vi "compressor_getenablstate.vi"(0 "CompressorDevRef":T1={"DevStatus"={"status"=FALSE, "code"=0, "source"=""}, "DigitalInputDevRef"={"DevStatus"={"status"=FALSE, "code"=0, "source"=""}, "DIO Channel"=enum."DIO 1", "Digital Module"=enum."Digital Module 1"}, "RelayDevRef"={"DevStatus"={"status"=FALSE, "code"=0, "source"=""}, "Relay Channel"=enum."Invalid", "Digital Module"=enum."Digital Module 1", "Relay Direction"=enum."Both directions"}}, 11 "error in (no error)":errorcluster) -> (4 "CompressorDevRef":T1={"DevStatus"={"status"=FALSE, "code"=0, "source"=""}, "DigitalInputDevRef"={"DevStatus"={"status"=FALSE, "code"=0, "source"=""}, "DIO Channel"=enum."DIO 1", "Digital Module"=enum."Digital Module 1"}, "RelayDevRef"={"DevStatus"={"status"=FALSE, "code"=0, "source"=""}, "Relay Channel"=enum."Invalid", "Digital Module"=enum."Digital Module 1", "Relay Direction"=enum."Both directions"}}, 6 "Enabled":bool, 10 "Compressor Running":bool, 12 "On/Off":bool, 13 "Charging":bool, 14 "Full":bool, 15 "error out":errorcluster)   [LabVIEW 2013]
doc: "Returns the enable/start state of the compressor and the on/off state of the compressor relay.\n\nThis software is licensed. Open the labview\\readme\\WPI Robotics Library Open Source License.txt file for more information."
uses:
  <vilib>/Rock Robotics/WPI/Compressor/WPI_CompressorDevRef.ctl
  <vilib>/Rock Robotics/WPI/DigitalInput/WPI_DigitalInputDevRef.ctl
  <vilib>/Rock Robotics/SystemInterfaces/DIO/FPGA_DIOChannel.ctl
  <vilib>/Rock Robotics/SystemInterfaces/Typedef/FPGA_TypedefDigitalModule.ctl
  <vilib>/Rock Robotics/WPI/Relay/WPI_RelayDevRef.ctl
  <vilib>/Rock Robotics/SystemInterfaces/DIO/FPGA_DIORelayChannel.ctl
  <vilib>/Rock Robotics/WPI/Relay/WPI_RelayDirection.ctl
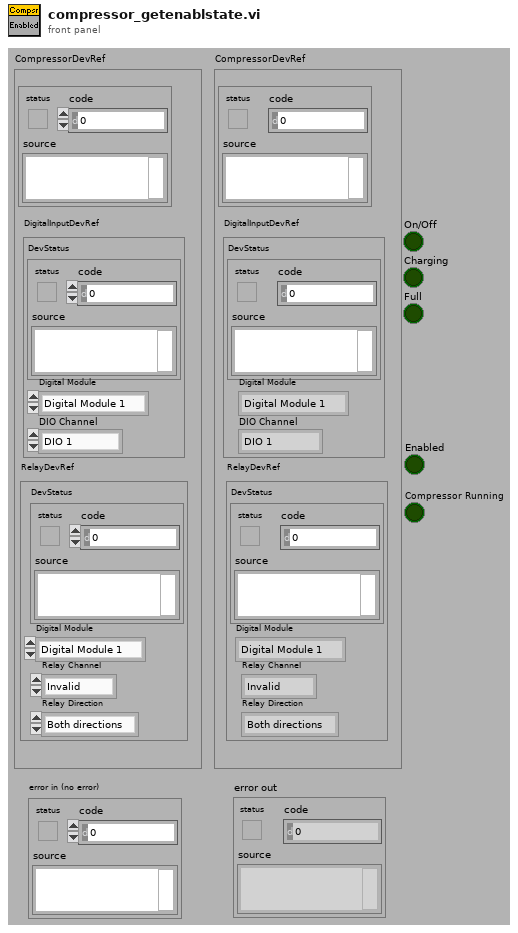
[diagram p1: front panel]
types:
  T1 = typedef "WPI_CompressorDevRef.ctl" = cluster{"DevStatus":errorcluster, "DigitalInputDevRef":T2, "RelayDevRef":T5}
  T2 = typedef "WPI_DigitalInputDevRef.ctl" = cluster{"DevStatus":errorcluster, "DIO Channel":T3, "Digital Module":T4}
  T3 = typedef "FPGA_DIOChannel.ctl" = enum8{"DIO 1", "DIO 2", "DIO 3", "DIO 4", "DIO 5", "DIO 6", "DIO 7", "DIO 8", "DIO 9", "DIO 10", "DIO 11", "DIO 12", "DIO 13", "DIO 14", "Invalid"}
  T4 = typedef "FPGA_TypedefDigitalModule.ctl" = enum16{"Digital Module 1", "Digital Module 2"}
  T5 = typedef "WPI_RelayDevRef.ctl" = cluster{"DevStatus":errorcluster, "Relay Channel":T6, "Digital Module":T4, "Relay Direction":T7}
  T6 = typedef "FPGA_DIORelayChannel.ctl" = enum8{"Relay 1", "Relay 2", "Relay 3", "Relay 4", "Relay 5", "Relay 6", "Relay 7", "Relay 8", "Invalid"}
  T7 = typedef "WPI_RelayDirection.ctl" = enum16{"Both directions", "Forward only", "Reverse only"}
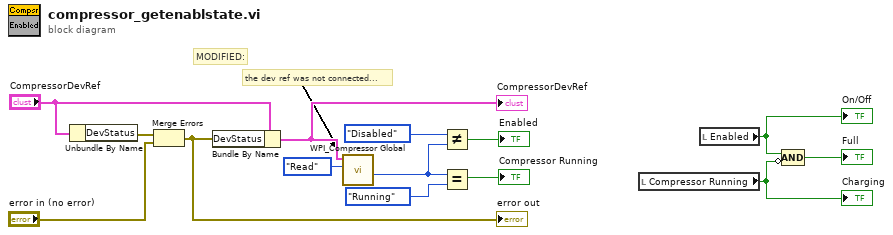
[diagram p0: block diagram]
diagram:
  # "the dev ref was not connected..."
  # "MODIFIED:"
  n1 = Unbundle By Name("CompressorDevRef") -> ("DevStatus"=w9:errorcluster)
  n2 = Merge Errors(w9, "error in (no error)") -> (w7:errorcluster)
  "error out" <- w7
  n3 = Bundle By Name(cluster="CompressorDevRef", "DevStatus"=w7) -> (w4:T1)
  "CompressorDevRef" <- w4
  n4 = call <vilib>:"WPI_Compressor Global.vi"("Operation"=enum16{"Read", "Write", "Add", "Remove"}."Read", "CompressorDevRef"=w4) -> ("Compressor State Out"=w5:enum16{"Disabled", "Running", "At Pressure"})  [unwired: 8 in, 1 out]
  n5 = Not Equal?(x=enum16{"Disabled", "Running", "At Pressure"}."Disabled" ("Compressor State"), y=w5) -> (x != y?=→"Enabled":bool)
  n6 = Equal?(x=w5, y=enum16{"Disabled", "Running", "At Pressure"}."Running" ("Compressor State")) -> (x = y?=→"Compressor Running":bool)
  n7 = local read "Compressor Running"() -> (w1:bool)
  "Charging" <- w1
  n8 = local read "Enabled"() -> (w2:bool)
  "On/Off" <- w2
  n9 = Compound Arithmetic op=AND(w2, invert w1) -> (→"Full":bool)
